vi "Pen.vi"(4 "Edge color":u32(colorbox), 6 "Fill color":u32(colorbox), 8 "error in (no error)":errorcluster, 9 "Current color (T)":u32(colorbox)=16777216, 10 "point(x,y)":cluster{"x":i16, "y":i16}, 11 "Tools Paint in":refnum<class "Tools Paint.lvclass">) -> (0 "error out":errorcluster, 2 "new picture":picture, 3 "Tools Paint out":refnum<class "Tools Paint.lvclass">, 5 "Current line color":u32(colorbox))   [LabVIEW 2020, in "Tools Paint.lvclass"]
uses:
  Tools Paint.lvclass
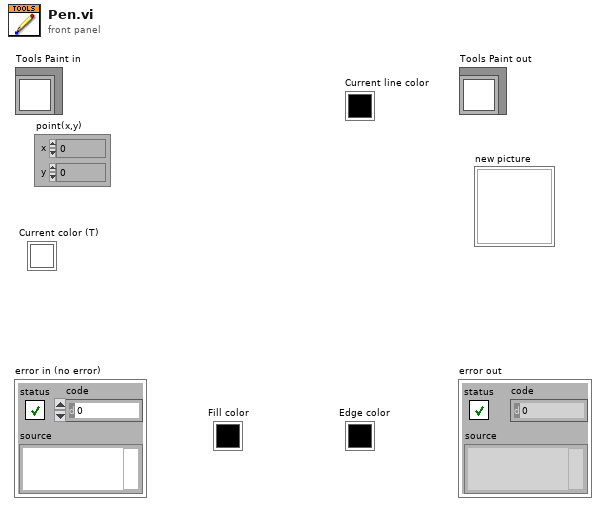
[diagram p1: front panel]
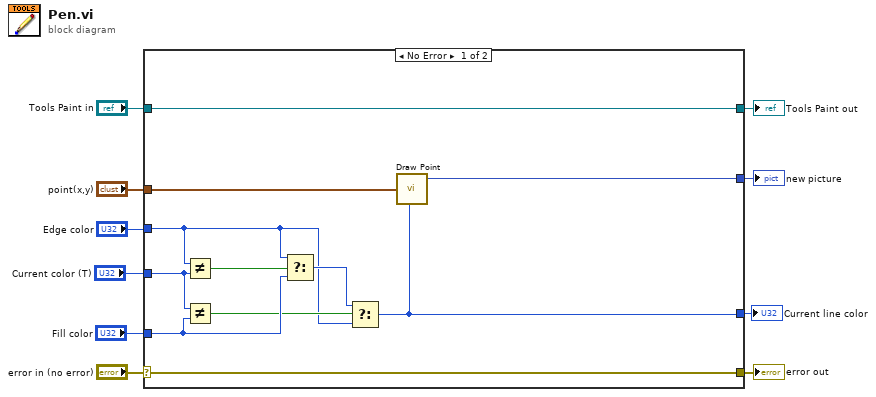
[diagram p0: block diagram]
diagram:
  n1 = case shown="No Error" "error in (no error)" {
    selector: "error in (no error)" -> [w20 w23]
    tunnel: [w20 w23] -> w9
    tunnel: [w21 w22] -> w7
    tunnel: "Tools Paint in" -> [w21 w22]
    tunnel: [w19 _] -> w6
    tunnel: "point(x,y)" -> [w18 _]
    tunnel: "Edge color" -> [w12 _]
    tunnel: "Current color (T)" -> [w17 _]
    tunnel: "Fill color" -> [w16 _]
    tunnel: [w11 _] -> w1
    frame No Error {
      n2 = Not Equal?(x=w12, y=w17) -> (x != y?=w14:bool)
      n3 = Not Equal?(x=w17, y=w16) -> (x != y?=w15:bool)
      n4 = Select(t=w12, s=w14, f=w16) -> (s? t:f=w13:u32)
      n5 = Select(t=w13, s=w15, f=w12) -> (s? t:f=w11:u32)
      n6 = call <vilib>:"Draw Point.vi"("point(x,y)"=w18, "color(black)"=w11) -> ("new picture"=w19:picture)  [unwired: 2 in, 5 out]
    }
    frame Error {
    }
  }
  "error out" <- w9
  "Tools Paint out" <- w7
  "new picture" <- w6
  "Current line color" <- w1
